vi "Connect.vi"(11 "OPC UA ENDpoint":string) -> (0 "error out":errorcluster, 1 "Success":bool, 2 "namespaces":string, 3 "session out":refnum<k35>)   [LabVIEW 2019]
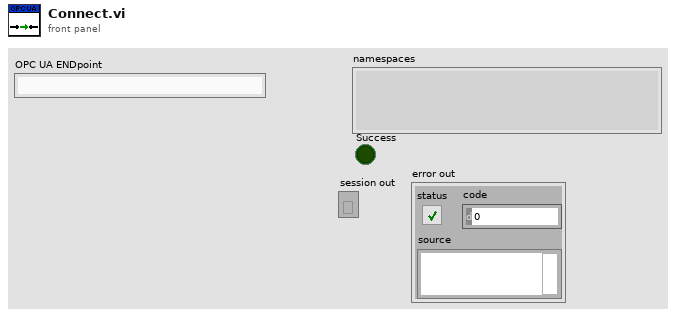
[diagram p1: front panel]
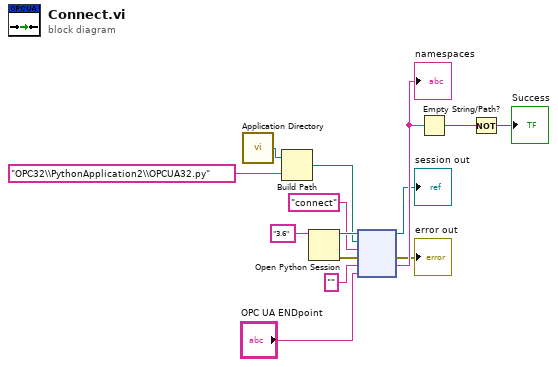
[diagram p0: block diagram]
diagram:
  n1 = call <vilib>:"Application Directory.vi"() -> ("Application Directory"=w3:path)
  n2 = Build Path(base path=w3, name or relative path="OPC32\\PythonApplication2\\OPCUA32.py") -> (appended path=w1:path)
  n3 = Open Python Session(python version="3.6" ("Python version")) -> (session out=w13:refnum<k35>, error out=w11:errorcluster)  [unwired: 2 in]
  n4 = node(w13, w1, "connect" ("function name"), w11, "", "OPC UA ENDpoint") -> (→"session out":refnum<k35>, →"error out":errorcluster, w9:string)  [unwired: 1 in, 2 out]
  "namespaces" <- w9
  n5 = Empty String/Path?(string/path=w9) -> (empty?=w8:bool)
  n6 = Not(x=w8) -> (.not. x?=→"Success":bool)
